vi "Set State.vi"(8 "error in (no error)":errorcluster, 10 "Output":T1, 11 "Inst.RP100 in":refnum<class "Inst.RP100.lvclass">) -> (0 "error out":errorcluster, 3 "Inst.RP100 out":refnum<class "Inst.RP100.lvclass">)   [LabVIEW 2019, in "Inst.RP100.lvclass"]
doc: "Set the output <b>Level</b> with <b>Slew</b> rate on the selected <b>Output Channel</b>"
uses:
  Inst.RP100.lvclass
  Typedefs/Output State--Enum.ctl
  Typedefs/Inst.RP100.PublicCommands--Enum.ctl
  Typedefs/setOutput--Cluster.ctl
  bd6c3626-3ffe-41a5-babe-17ac00828b50.vi
  bd6c3626-3ffe-41a5-babe-17ac00828b50.vi/4b8c8db5-530d-4966-b0d6-d81441259936.vi
  bd6c3626-3ffe-41a5-babe-17ac00828b50.vi/4b8c8db5-530d-4966-b0d6-d81441259936.vi/53ae95df-1a2e-490d-9a8c-97a716d3083e.vi
  bd6c3626-3ffe-41a5-babe-17ac00828b50.vi/4b8c8db5-530d-4966-b0d6-d81441259936.vi/818eca58-ac9c-45b6-8e1e-8442631c0f81.vi
  <vilib>/Utility/Data Type/Get Type Information.vi
  <vilib>/JDP Science/JSONtext/JSON text to Variant.vi
  <vilib>/JDP Science/JSONtext/LVClass Serializer/JSONtext LVClass Serializer.lvclass
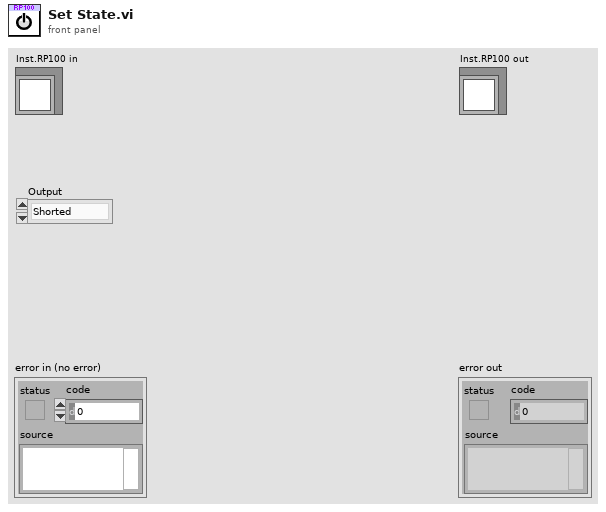
[diagram p1: front panel]
types:
  T1 = typedef "Inst.RP100.lvclass/Output State--Enum.ctl" = enum16{"Shorted", "Enabled"}
  T2 = typedef "Inst.RP100.lvclass/setOutput--Cluster.ctl" = cluster{"State":T1}
  T3 = typedef "Inst.RP100.lvclass/Inst.RP100.PublicCommands--Enum.ctl" = enum16{"setState", "setStrain", "getStrain", "setLevel", "getLevel"}
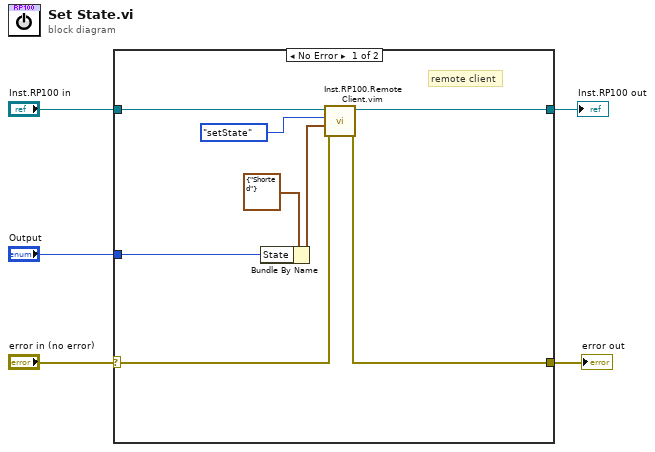
[diagram p0: block diagram]
diagram:
  n1 = case shown="No Error" "error in (no error)" {
    selector: "error in (no error)" -> [w11 w15]
    tunnel: [w10 w15] -> w4
    tunnel: "Output" -> [w7 _]
    tunnel: "Inst.RP100 in" -> [w13 w14]
    tunnel: [w12 w14] -> w1
    frame No Error {
      # "remote client"
      n2 = Bundle By Name(cluster=T2 {"State"=enum."Shorted"} ("setOutput"), "State"=w7) -> (w8:T2)
      n3 = call "Inst.RP100.Remote Client.vim"("error in (no error)"=w11, "params"=w8, "Commands"=Inst.RP100.PublicCommands--Enum."setState", "Inst.RP100 in"=w13) -> ("error out"=w10:errorcluster, "Inst.RP100 out"=w12:refnum<class "Inst.RP100.lvclass">)  [unwired: 5 in, 1 out]
    }
    frame Error {
    }
  }
  "error out" <- w4
  "Inst.RP100 out" <- w1
